vi "niDTS BT Rx Test UTIL EDR Parameters to BT RX Parameters.vi"(7 "BT EDR Parameters":T1={"Channel"=3, "Tx Power (dBm)"=0.0, "External Attenuation (dB)"=0.0, "EDR Packet type"=enum."DH1", "Data Rate (bits/symbol)"=2, "Payload Data"=enum."PN9", "Carrier Mode"=enum."Burst", "Number of Packets"=1500, "Report Period (ms)"=1000.0, "BD ADDRESS"="", "Dirty Packets"=FALSE, "Corrupt Alternate CRC"=FALSE, "Packet Header"={"LT Address"=0, "Flow"=0, "ARQN"=enum."NAK", "Sequence Bit"=0}, "Payload Header"={"LCh"=0, "HeaderFlowControlBit"=FALSE, "Length (-1 AutoSet Max)"=-1}, "Trigger"={"TriggerEdge"=enum."RISing", "TriggerSource"=enum."IMMediate", "TriggerDelay (sec)"=0.0, "TriggerTimeout (sec)"=0.0}}) -> (8 "BT Rx Parameters":T8={"Channel"=3, "Dut Tx Power"=0.0, "External Attenuation (dB)"=[0.0], "Data Rate"=enum."2", "Packet type"=enum."DH1", "Payload Data"=enum."PN9", "Carrier Mode"=enum."Burst", "Number of Packets"=1500, "Report Period (ms)"=1000.0, "BD ADDRESS"=0, "Dirty Tx"=FALSE, "Corrupt Alternate CRC"=FALSE, "Packet Header"={"LT Address"=0, "Flow"=0, "ARQN"=enum."NAK", "Sequence Bit"=0}, "Payload Header"={"LCh"=0, "HeaderFlowControlBit"=FALSE, "Length (-1 AutoSet Max)"=-1}, "Trigger"={"TriggerEdge"=enum."RISing", "TriggerSource"=enum."RTSI 0", "TriggerDelay (sec)"=0.0, "TriggerTimeout (sec)"=0.0}} {"BD ADDRESS" max=16777215 format="%.0x"})   [LabVIEW 2015, in "niDTS BT.lvlib"]
uses:
  niDTS BT.lvlib
  Rx Test/Includes/niDTS BT Rx Test INC Parameters.ctl
  Includes/niDTS BT INC Packet Type.ctl
  Tx Test/Includes/niDTS BT Tx Test INC BD Payload Data.ctl
  Rx Test/Includes/niDTS BT Rx Test INC Carrier Mode.ctl
  Rx Test/Includes/niDTS BT Rx Test INC Packet Header.ctl
  Rx Test/Includes/niDTS BT Rx Test INC Payload Header.ctl
  Includes/niDTS BT DUT INC SG Trigger.ctl
  Includes/niDTS BT EDR Rx Test INC Parameters.ctl
  BDR Tx Test/Includes/niDTS BT INC BDR Packet Type.ctl
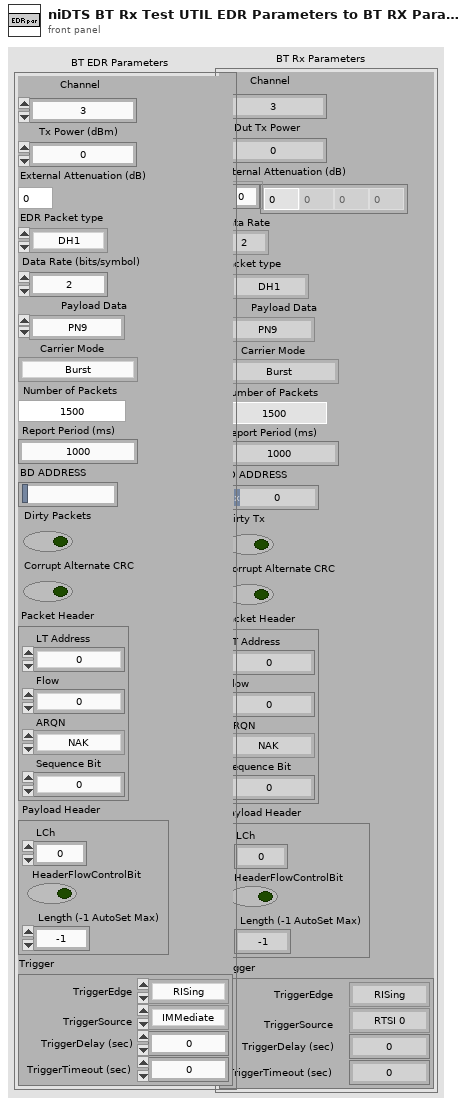
[diagram p1: front panel]
types:
  T1 = typedef "niDTS BT.lvlib/niDTS BT EDR Rx Test INC Parameters.ctl" = cluster{"Channel":i32, "Tx Power (dBm)":dbl, "External Attenuation (dB)":dbl, "EDR Packet type":T2, "Data Rate (bits/symbol)":i32, "Payload Data":T3, "Carrier Mode":T4, "Number of Packets":i32, "Report Period (ms)":dbl, "BD ADDRESS":string, "Dirty Packets":bool, "Corrupt Alternate CRC":bool, "Packet Header":T5, "Payload Header":T6, "Trigger":T7}
  T2 = typedef "niDTS BT.lvlib/niDTS BT INC BDR Packet Type.ctl" = enum16{"NULL", "POLL", "FHS", "DM1", "DH1", "HV1", "HV2", "HV3", "EV3", "DV", "AUX1", "DM3", "DH3", "EV4", "EV5", "DM5", "DH5"}
  T3 = typedef "niDTS BT.lvlib/niDTS BT Tx Test INC BD Payload Data.ctl" = enum16{"0", "1", "01", "00001111", "PN9", "AUTO"}
  T4 = typedef "niDTS BT.lvlib/niDTS BT Rx Test INC Carrier Mode.ctl" = enum16{"Burst", "Continuous"}
  T5 = typedef "niDTS BT.lvlib/niDTS BT Rx Test INC Packet Header.ctl" = cluster{"LT Address":i8, "Flow":i8, "ARQN":enum16{"NAK", "ACK"}, "Sequence Bit":i8}
  T6 = typedef "niDTS BT.lvlib/niDTS BT Rx Test INC Payload Header.ctl" = cluster{"LCh":i32, "HeaderFlowControlBit":bool, "Length (-1 AutoSet Max)":i32}
  T7 = typedef "niDTS BT.lvlib/niDTS BT DUT INC SG Trigger.ctl" = cluster{"TriggerEdge":enum16{"RISing", "FALLing"}, "TriggerSource":enum16{"IMMediate", "PFI 0", "PFI 1", "RTSI 0", "RTSI 1", "RTSI 2", "RTSI 3", "RTSI 4", "RTSI 5", "RTSI 6", "RTSI 7", "PXI STAR", "Software"}, "TriggerDelay (sec)":dbl, "TriggerTimeout (sec)":dbl}
  T8 = typedef "niDTS BT.lvlib/niDTS BT Rx Test INC Parameters.ctl" = cluster{"Channel":i32, "Dut Tx Power":dbl, "External Attenuation (dB)":dbl[], "Data Rate":enum16{"1", "2", "3"}, "Packet type":T9, "Payload Data":T3, "Carrier Mode":T4, "Number of Packets":i32, "Report Period (ms)":dbl, "BD ADDRESS":i64, "Dirty Tx":bool, "Corrupt Alternate CRC":bool, "Packet Header":T5, "Payload Header":T6, "Trigger":T7}
  T9 = typedef "niDTS BT.lvlib/niDTS BT INC Packet Type.ctl" = enum16{"NULL", "POLL", "FHS", "DM1", "DH1", "HV1", "HV2", "HV3", "EV3", "DV", "AUX1", "DM3", "DH3", "EV4", "EV5", "DM5", "DH5", "LE-TP"}
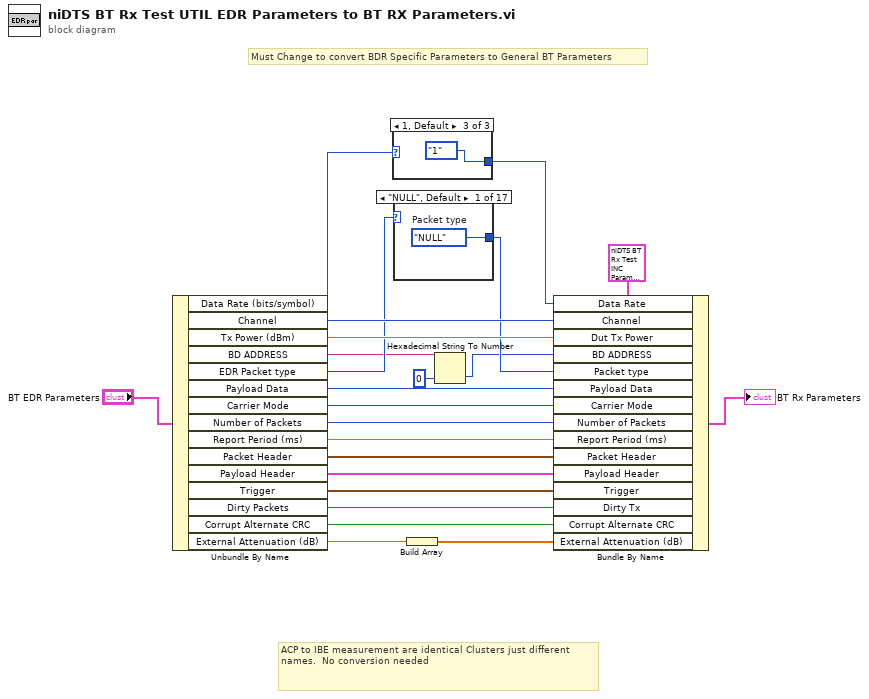
[diagram p0: block diagram]
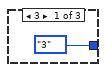
[diagram p2: hidden frame]
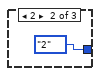
[diagram p3: hidden frame]
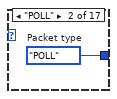
[diagram p4: hidden frame]
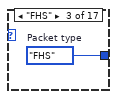
[diagram p5: hidden frame]
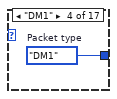
[diagram p6: hidden frame]
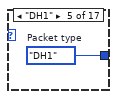
[diagram p7: hidden frame]
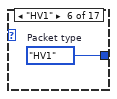
[diagram p8: hidden frame]
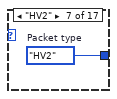
[diagram p9: hidden frame]
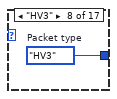
[diagram p10: hidden frame]
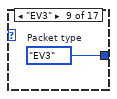
[diagram p11: hidden frame]
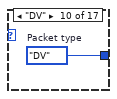
[diagram p12: hidden frame]
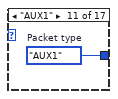
[diagram p13: hidden frame]
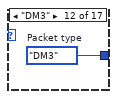
[diagram p14: hidden frame]
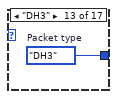
[diagram p15: hidden frame]
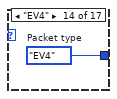
[diagram p16: hidden frame]
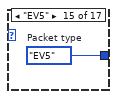
[diagram p17: hidden frame]
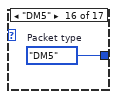
[diagram p18: hidden frame]
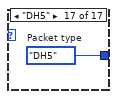
[diagram p19: hidden frame]
diagram:
  # "ACP to IBE measurement are identical Clusters just different names.  No conversion needed"
  # "Must Change to convert BDR Specific Parameters to General BT Parameters"
  n1 = Unbundle By Name("BT EDR Parameters") -> ("Data Rate (bits/symbol)"=w3:i32, "Channel"=w21:i32, "Tx Power (dBm)"=w20:dbl, "BD ADDRESS"=w7:string, "EDR Packet type"=w19:T2, "Payload Data"=w18:T3, "Carrier Mode"=w17:T4, "Number of Packets"=w16:i32, "Report Period (ms)"=w15:dbl, "Packet Header"=w14:T5, "Payload Header"=w13:T6, "Trigger"=w10:T7, "Dirty Packets"=w6:bool, "Corrupt Alternate CRC"=w5:bool, "External Attenuation (dB)"=w2:dbl)
  n2 = case shown="1, Default" w3 {
    tunnel: [enum16{"1", "2", "3"}."3" ("Data Rate") enum16{"1", "2", "3"}."2" ("Data Rate") enum16{"1", "2", "3"}."1" ("Data Rate")] -> w4
    frame 3 {
    }
    frame 2 {
    }
    frame 1, Default {
    }
  }
  n3 = case shown="\"NULL\", Default" w19 {
    tunnel: [w27 w28 w29 w30 w31 w32 w33 w34 w35 w36 w37 w38 w39 w40 w41 w42 w43] -> w12
    frame "NULL", Default {
      w27 = niDTS_BT_INC_Packet_Type."NULL"  # Packet type
    }
    frame "POLL" {
      w28 = niDTS_BT_INC_Packet_Type."POLL"  # Packet type
    }
    frame "FHS" {
      w29 = niDTS_BT_INC_Packet_Type."FHS"  # Packet type
    }
    frame "DM1" {
      w30 = niDTS_BT_INC_Packet_Type."DM1"  # Packet type
    }
    frame "DH1" {
      w31 = niDTS_BT_INC_Packet_Type."DH1"  # Packet type
    }
    frame "HV1" {
      w32 = niDTS_BT_INC_Packet_Type."HV1"  # Packet type
    }
    frame "HV2" {
      w33 = niDTS_BT_INC_Packet_Type."HV2"  # Packet type
    }
    frame "HV3" {
      w34 = niDTS_BT_INC_Packet_Type."HV3"  # Packet type
    }
    frame "EV3" {
      w35 = niDTS_BT_INC_Packet_Type."EV3"  # Packet type
    }
    frame "DV" {
      w36 = niDTS_BT_INC_Packet_Type."DV"  # Packet type
    }
    frame "AUX1" {
      w37 = niDTS_BT_INC_Packet_Type."AUX1"  # Packet type
    }
    frame "DM3" {
      w38 = niDTS_BT_INC_Packet_Type."DM3"  # Packet type
    }
    frame "DH3" {
      w39 = niDTS_BT_INC_Packet_Type."DH3"  # Packet type
    }
    frame "EV4" {
      w40 = niDTS_BT_INC_Packet_Type."EV4"  # Packet type
    }
    frame "EV5" {
      w41 = niDTS_BT_INC_Packet_Type."EV5"  # Packet type
    }
    frame "DM5" {
      w42 = niDTS_BT_INC_Packet_Type."DM5"  # Packet type
    }
    frame "DH5" {
      w43 = niDTS_BT_INC_Packet_Type."DH5"  # Packet type
    }
  }
  n4 = Build Array(w2) -> (w1:dbl[])
  n5 = Hexadecimal String To Number(string=w7, default (0uL)=i64 0 ("default (0 U32)")) -> (number=w8:i64)  [unwired: 1 in, 1 out]
  n6 = Bundle By Name(cluster=T8 {"Channel"=0, "Dut Tx Power"=0.0, "External Attenuation (dB)"=[0.0], "Data Rate"=enum."3", "Packet type"=enum."DH1", "Payload Data"=enum."PN9", "Carrier Mode"=enum."Burst", "Number of Packets"=0, "Report Period (ms)"=0.0, "BD ADDRESS"=12329017, "Dirty Tx"=FALSE, "Corrupt Alternate CRC"=FALSE, "Packet Header"={"LT Address"=0, "Flow"=0, "ARQN"=enum."NAK", "Sequence Bit"=0}, "Payload Header"={"LCh"=0, "HeaderFlowControlBit"=FALSE, "Length (-1 AutoSet Max)"=0}, "Trigger"={"TriggerEdge"=enum."RISing", "TriggerSource"=enum."IMMediate", "TriggerDelay (sec)"=0.0, "TriggerTimeout (sec)"=0.0}} ("Parameters 2"), "Data Rate"=w4, "Channel"=w21, "Dut Tx Power"=w20, "BD ADDRESS"=w8, "Packet type"=w12, "Payload Data"=w18, "Carrier Mode"=w17, "Number of Packets"=w16, "Report Period (ms)"=w15, "Packet Header"=w14, "Payload Header"=w13, "Trigger"=w10, "Dirty Tx"=w6, "Corrupt Alternate CRC"=w5, "External Attenuation (dB)"=w1) -> (→"BT Rx Parameters":T8)
